vi "3d array testMOD1PlaneFill.vi"() -> ()   [LabVIEW 2011]
panel:
  in  "Stop Button":bool
  out "Intensity Slice":sgl[][](array[numeric])
  out "Array 3D":sgl[][][](array[numeric])
  in  "XY Plot Depth":u16(ring) items=["0", "1", "2", "3", "4"]
  in  "Plot":u16(ring) items=["XY", "X cross", "Y cross"]
  out "Intensity Graph":sgl[][](graph)
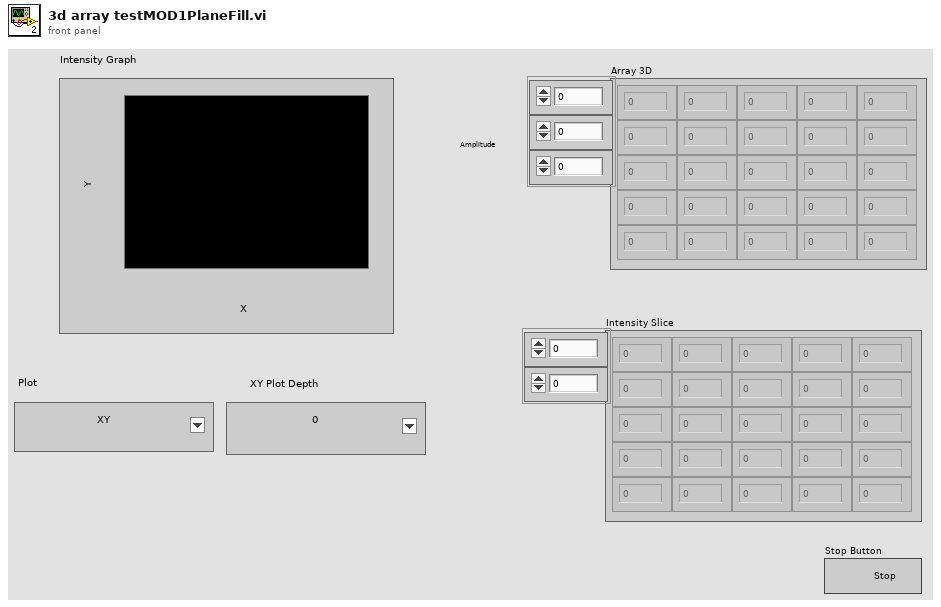
[diagram p1: front panel]
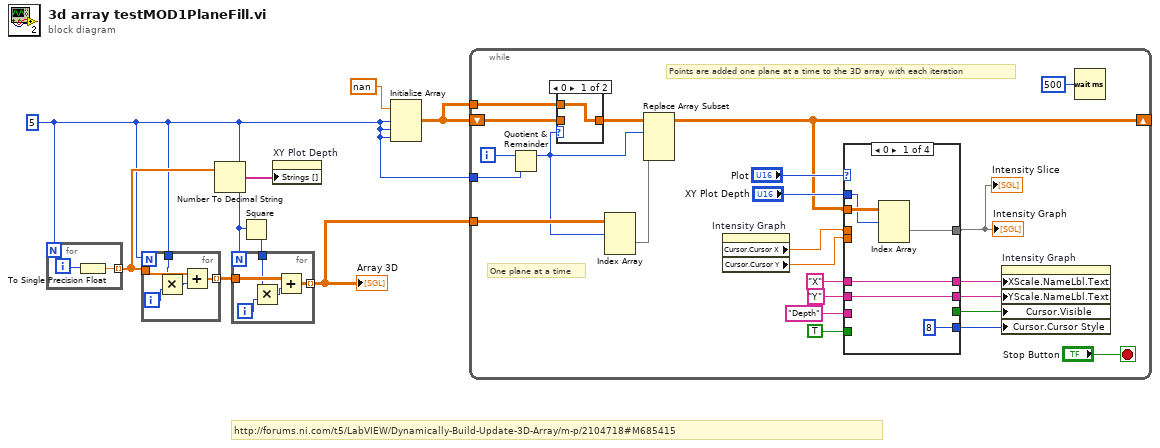
[diagram p0: block diagram]
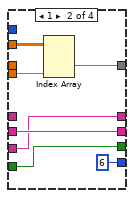
[diagram p2: hidden frame]
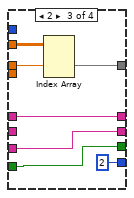
[diagram p3: hidden frame]
diagram:
  w4 = 5
  # "http://forums.ni.com/t5/LabVIEW/Dynamically-Build-Update-3D-Array/m-p/2104718#M685415"
  n1 = for {
    N: w4 -> [_]
    tunnel: [w10] -> w7 mode=indexing
    i -> [w9]
    n2 = To Single Precision Float(number=w9) -> (single precision float=w10:sgl)
  }
  n3 = for {
    N: w4 -> [_]
    tunnel: [w14] -> w6 mode=indexing
    tunnel: w7 -> [w15]
    tunnel: w4 -> [w11]
    i -> [w13]
    n4 = Multiply(x=w11, y=w13) -> (x*y=w12:i32)
    n5 = Add(x=w15, y=w12) -> (x+y=w14:sgl[])
  }
  n6 = Number To Decimal String(number=w7) -> (decimal integer string=w8:string[])  [unwired: 1 in]
  n7 = Square(x=w4) -> (x^2=w2:i32)
  n8 = for {
    N: w4 -> [_]
    tunnel: w6 -> [w20]
    tunnel: [w19] -> w1 mode=indexing
    tunnel: w2 -> [w17]
    i -> [w18]
    n9 = Multiply(x=w17, y=w18) -> (x*y=w16:i32)
    n10 = Add(x=w20, y=w16) -> (x+y=w19:sgl[][])
  }
  "Array 3D" <- w1
  n11 = property on="XY Plot Depth" class="Ring (strict)"("Strings []"=w8) -> ()  [unwired: 2 in, 2 out]
  n12 = Initialize Array(sgl nan ("element"), w4, w4, w4) -> (w3:sgl[][][])
  n13 = while {
    shift-right: [w24] -> _
    shift-left: w3 -> [w39]
    tunnel: w4 -> [w36]
    tunnel: w1 -> [w42]
    tunnel: w3 -> [w38]
    i -> [w37]
    stop <- "Stop Button" stop-if-true
    # "One plane at a time"
    # "Points are added one plane at a time to the 3D array with each iteration"
    n14 = Quotient & Remainder(x=w37, y=w36) -> (x-y*floor(x/y)=w35:i32)  [unwired: 1 out]
    n15 = case shown="0" w35 {
      tunnel: [w65 w66] -> w40
      tunnel: w39 -> [_ w66]
      tunnel: w38 -> [w65 _]
      frame 0 {
      }
      frame Default {
      }
    }
    n16 = Index Array(array=w42, index (dim 0)=w35) -> (element=w41:sgl[][])  [unwired: 2 in]
    n17 = Replace Array Subset(array=w40, new element=w41, index (dim 0)=w35) -> (w24:sgl[][][])  [unwired: 2 in]
    n18 = property on="Intensity Graph" class="IntGraph (strict)"() -> ("Cursor.Cursor X"=w23:dbl, "Cursor.Cursor Y"=w22:dbl)  [unwired: 2 in, 2 out]
    n19 = case shown="0" "Plot" {
      tunnel: w24 -> [w50 w57 w64 _]
      tunnel: [w49 w56 w63 _] -> w21
      tunnel: "XY Plot Depth" -> [w46 _ _ _]
      tunnel: [w48 w54 w60 _] -> w34
      tunnel: w23 -> [_ _ w61 _]
      tunnel: w22 -> [_ w53 _ _]
      tunnel: [w47 w55 w62 _] -> w33
      tunnel: "X" ("X Scale.Name Label.Text") -> [w48 _ w60 _]
      tunnel: "Y" ("X Scale.Name Label.Text") -> [w47 w55 _ _]
      tunnel: "Depth" ("Y Scale.Name Label.Text") -> [_ w54 w62 _]
      tunnel: [u8 8 ("Cursor.Cursor Style") u8 6 ("Cursor.Cursor Style") u8 2 ("Cursor.Cursor Style") _] -> w29
      tunnel: [_ w51 w58 _] -> w28
      tunnel: TRUE -> [_ w51 w58 _]
      frame 0 {
        n20 = Index Array(array=w50, index (dim 0)=w46) -> (element=w49:sgl[][])  [unwired: 2 in]
      }
      frame 1 {
        n21 = Index Array(array=w57, index (dim 2)=w53) -> (element=w56:sgl[][])  [unwired: 2 in]
      }
      frame 2 {
        n22 = Index Array(array=w64, index (dim 1)=w61) -> (element=w63:sgl[][])  [unwired: 2 in]
      }
      frame Default {
      }
    }
    "Intensity Graph" <- w21
    "Intensity Slice" <- w21
    n23 = property on="Intensity Graph" class="IntGraph (strict)"("XScale.NameLbl.Text"=w34, "YScale.NameLbl.Text"=w33, "Cursor.Visible"=w28, "Cursor.Cursor Style"=w29) -> ()  [unwired: 2 in, 2 out]
    n24 = Wait (ms)(milliseconds to wait=u32 500) -> ()  [unwired: 1 out]
  }
